vi "Open PID Configuration.vi"(8 "Error In":errorcluster) -> (0 "Error Out":errorcluster, 2 "SP":dbl=0.55, 3 "PID Parameters":cluster{"Kp":dbl, "Ti [s]":dbl, "Td [s]":dbl}={"Kp"=0.55, "Ti [s]"=18.0, "Td [s]"=0.0})   [LabVIEW 2018]
uses:
  <vilib>/Utility/config.llb/Read Key (Double).vi
  <vilib>/Utility/config.llb/NI_LVConfig.lvlib
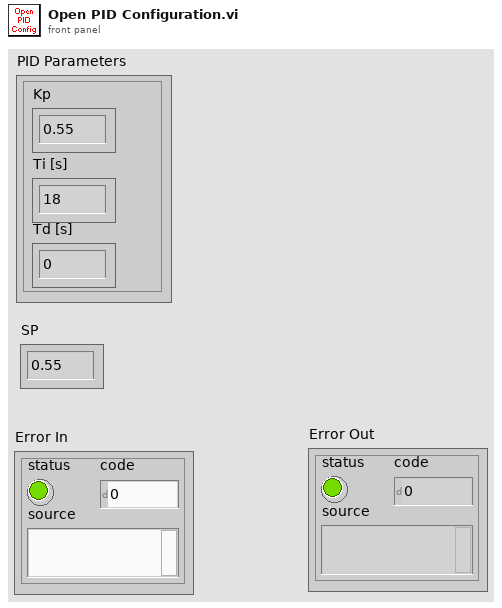
[diagram p1: front panel]
types:
  T1 = typedef "NI_LVConfig.lvlib/Config Data RefNum.ctl" = refnum<k1>
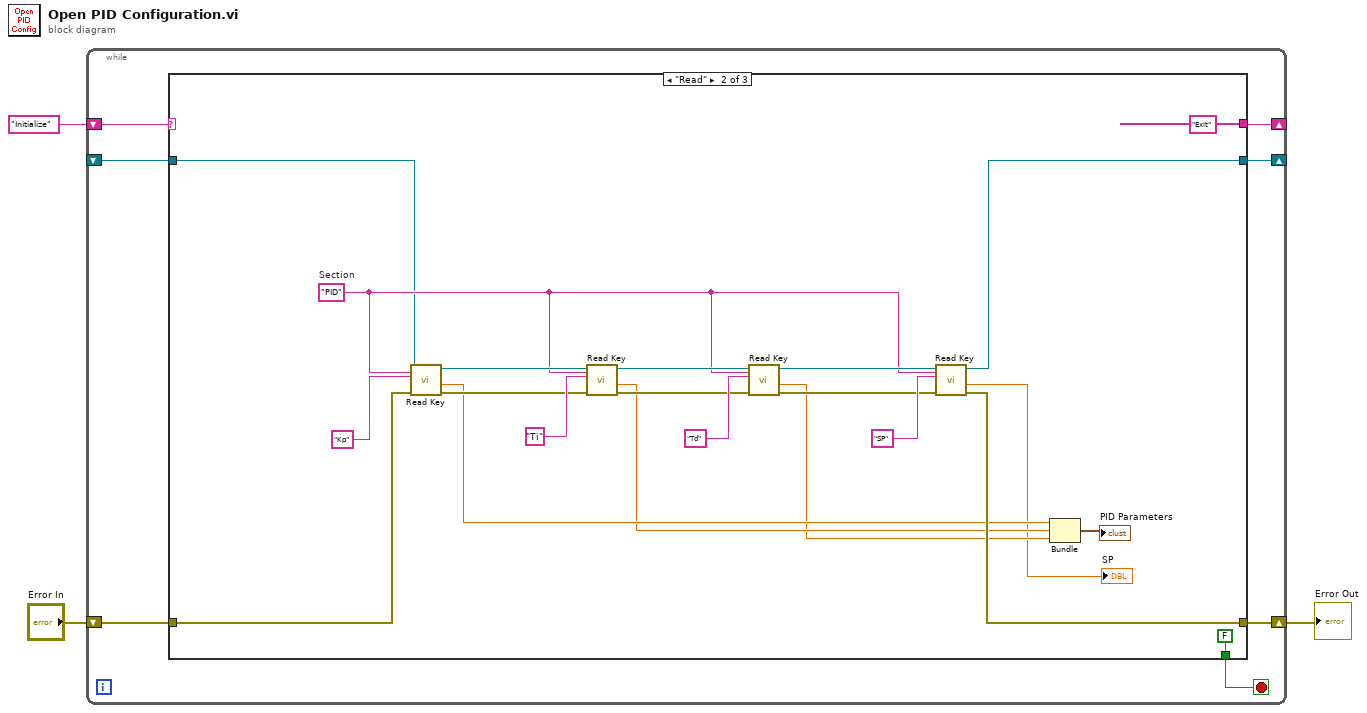
[diagram p0: block diagram]
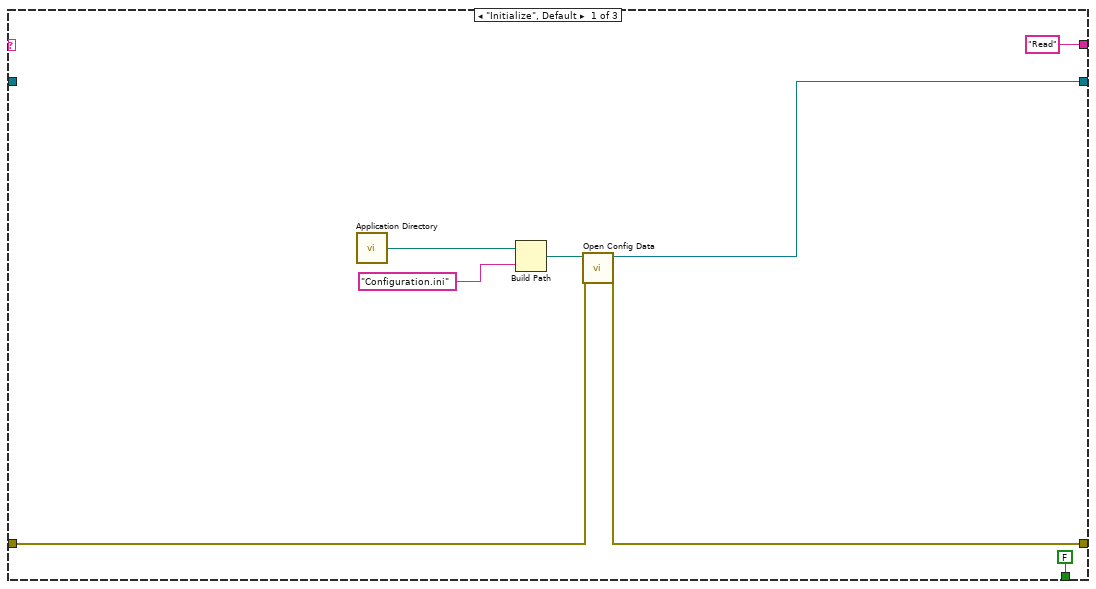
[diagram p2: hidden frame]
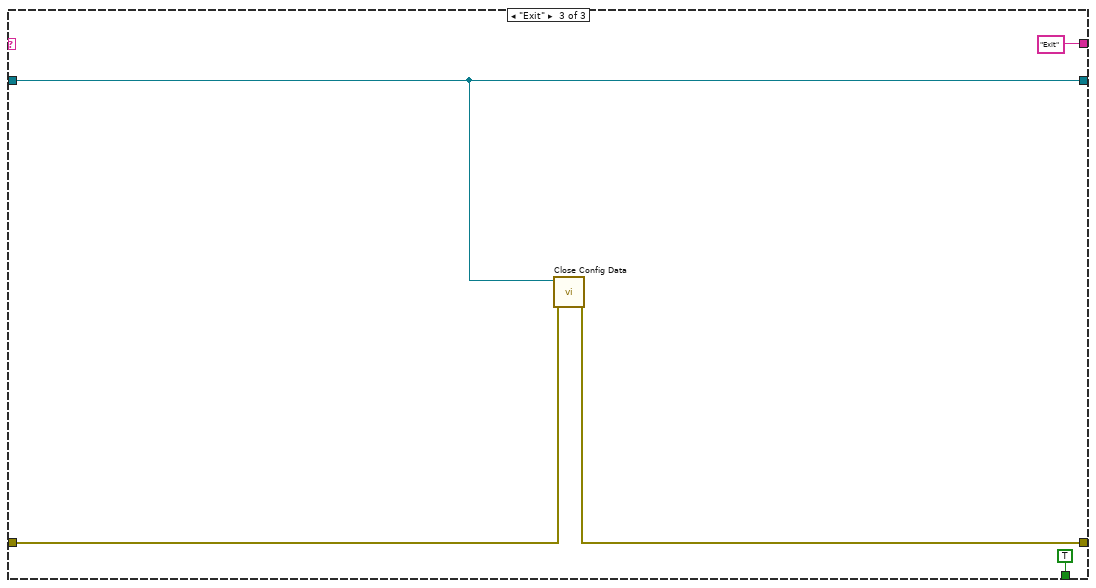
[diagram p3: hidden frame]
diagram:
  n1 = while {
    shift-right: [w6] -> _
    shift-left: "Initialize" ("key") -> [w10]
    shift-right: [w7] -> _
    shift-left: _ -> [w9]
    shift-right: [w4] -> w1
    shift-left: "Error In" -> [w8]
    stop <- w5 stop-if-true
    n2 = case shown="\"Read\"" w10 {
      tunnel: w9 -> [_ w25 w43]
      tunnel: w8 -> [w12 w27 w42]
      tunnel: [w13 w24 w43] -> w7
      tunnel: ["Read" ("key") "Exit" ("key") "Exit" ("key")] -> w6
      tunnel: [FALSE FALSE TRUE] -> w5
      tunnel: [w11 w26 w41] -> w4
      frame "Initialize", Default {
        n3 = call <vilib>:"Application Directory.vi"() -> ("Application Directory"=w16:path)
        n4 = Build Path(base path=w16, name or relative path="Configuration.ini") -> (appended path=w14:path)
        n5 = call <vilib>:"Open Config Data.vi"("error in (no error)"=w12, "configuration file path"=w14) -> ("error out"=w11:errorcluster, "refnum"=w13:T1)  [unwired: 7 in, 1 out]
      }
      frame "Read" {
        w28 = "PID"  # Section
        n6 = call-poly <vilib>:"Read Key.vi"("section"=w28, "error in (no error)"=w27, "key"="Kp", "refnum"=w25) -> ("error out"=w37:errorcluster, "value"=w23:dbl, "refnum out"=w36:T1)  [unwired: 4 in, 1 out]
        n7 = call-poly <vilib>:"Read Key.vi"("section"=w28, "error in (no error)"=w37, "key"="Ti", "refnum"=w36) -> ("error out"=w31:errorcluster, "value"=w22:dbl, "refnum out"=w32:T1)  [unwired: 4 in, 1 out]
        n8 = call-poly <vilib>:"Read Key.vi"("section"=w28, "error in (no error)"=w31, "key"="Td", "refnum"=w32) -> ("error out"=w29:errorcluster, "value"=w21:dbl, "refnum out"=w30:T1)  [unwired: 4 in, 1 out]
        n9 = call-poly <vilib>:"Read Key.vi"("section"=w28, "error in (no error)"=w29, "key"="SP", "refnum"=w30) -> ("error out"=w26:errorcluster, "value"=→"SP":dbl, "refnum out"=w24:T1)  [unwired: 4 in, 1 out]
        n10 = Bundle("value"=w23, "value"=w22, "value"=w21) -> (→"PID Parameters":cluster{"value":dbl, "value":dbl, "value":dbl})  [unwired: 1 in]
      }
      frame "Exit" {
        n11 = call <vilib>:"Close Config Data.vi"("error in (no error)"=w42, "refnum"=w43) -> ("error out"=w41:errorcluster)  [unwired: 8 in, 1 out]
      }
    }
  }
  "Error Out" <- w1
